vi "AngleToHCDIO.vi"(11 "Angle":dbl) -> (3 "Out":dbl)   [LabVIEW 2019]
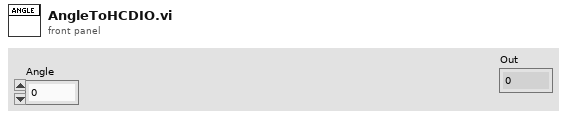
[diagram p1: front panel]
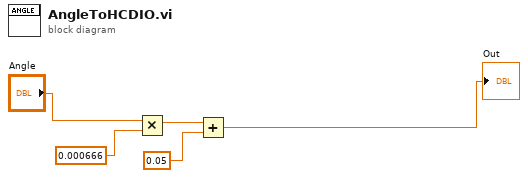
[diagram p0: block diagram]
diagram:
  n1 = Multiply(x="Angle", y=0.000666) -> (x*y=w3:dbl)
  n2 = Add(x=w3, y=0.05) -> (x+y=→"Out":dbl)
